vi "DigitalWrite.vi"(3 "error in (no error)":errorcluster, 4 "Value":bool, 5 "Terminal in":u8, 6 "VISA Refnum in":refnum<visa-resource-name>) -> (0 "error out":errorcluster, 1 "Return":u8[](array[numeric]), 2 "VISA Refnum out":refnum<visa-resource-name>)   [LabVIEW 2016]
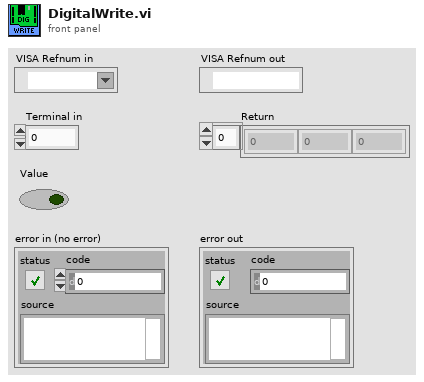
[diagram p1: front panel]
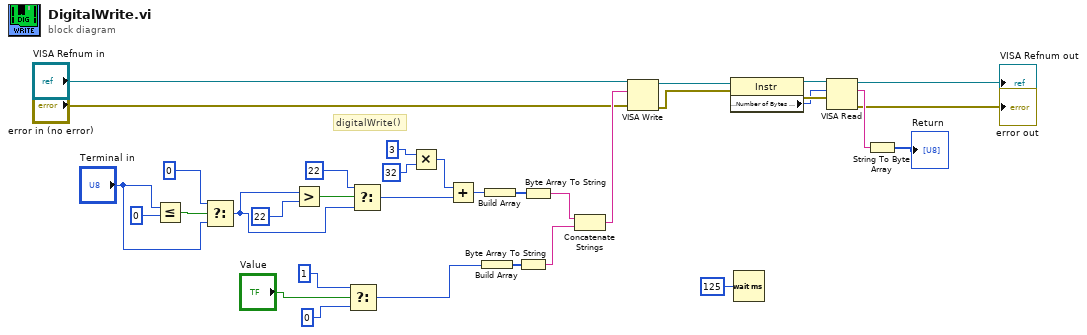
[diagram p0: block diagram]
diagram:
  # "digitalWrite()"
  n1 = Less Or Equal?(x="Terminal in", y=u8 0) -> (x <= y?=w17:bool)
  n2 = Select(t=u8 0, s=w17, f="Terminal in") -> (s? t:f=w20:u8)
  n3 = Greater?(x=w20, y=u8 22) -> (0:w12:bool)
  n4 = Select(t=u8 1, s="Value", f=u8 0) -> (s? t:f=w33:u8)
  n5 = Select(t=u8 22, s=w12, f=w20) -> (s? t:f=w34:u8)
  n6 = Multiply(x=u8 3, y=u8 32) -> (x*y=w15:u8)
  n7 = Add(x=w15, y=w34) -> (x+y=w21:u8)
  n8 = Build Array(w33) -> (w23:u8[])
  n9 = Build Array(w21) -> (w22:u8[])
  n10 = Byte Array To String(unsigned byte array=w23) -> (string=w24:string)
  n11 = Byte Array To String(unsigned byte array=w22) -> (string=w25:string)
  n12 = Concatenate Strings(w25, w24) -> (w26:string)
  n13 = VISA Write(VISA resource name="VISA Refnum in", write buffer=w26, error in (no error)="error in (no error)") -> (VISA resource name out=w5:refnum<visa-resource-name>, error out=w4:errorcluster)  [unwired: 1 out]
  n14 = property class="Instr"(reference=w5, error in=w4) -> (reference out=w8:refnum<visa-resource-name>, error out=w7:errorcluster, "Serial Settings:Number of Bytes at Serial Port"=w6:u32)
  n15 = Wait (ms)(milliseconds to wait=u32 125) -> ()  [unwired: 1 out]
  n16 = VISA Read(VISA resource name=w8, byte count=w6, error in (no error)=w7) -> (VISA resource name out=→"VISA Refnum out":refnum<visa-resource-name>, read buffer=w28:string, error out=→"error out":errorcluster)  [unwired: 1 out]
  n17 = String To Byte Array(string=w28) -> (unsigned byte array=→"Return":u8[])
